vi "control function to channels.vi"(11 "control module configuration":T1 {"output range"."output low" format="%.2f"; "output range"."output high" format="%.2f"}) -> (3 "channels":refnum<class "TBM channel.lvclass">[](array[class]))   [LabVIEW 2013, in "configuration tests.lvlib" / "TEST CONFIGURATION.lvclass"]
uses:
  TEST CONFIGURATION.lvclass
  <vilib>/NI/Tag Bus Module Framework/channel/TBM channel.lvclass
  control module configuration.ctl
  gains.ctl
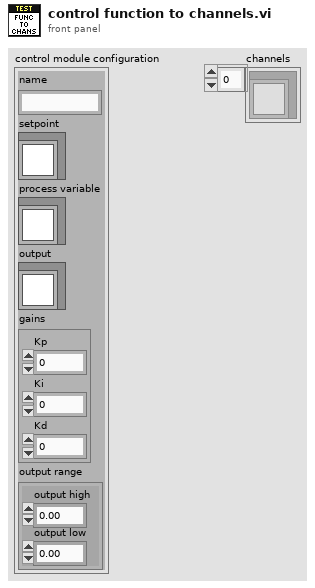
[diagram p1: front panel]
types:
  T1 = typedef "configuration tests.lvlib/TEST CONFIGURATION.lvclass/control module configuration.ctl" = cluster{"name":string, "setpoint":refnum<class "TBM channel.lvclass">, "process variable":refnum<class "TBM channel.lvclass">, "output":refnum<class "TBM channel.lvclass">, "gains":T2, "output range":cluster{"output high":dbl, "output low":dbl}}
  T2 = typedef "configuration tests.lvlib/TEST CONFIGURATION.lvclass/gains.ctl" = cluster{"Kp":dbl, "Ki":dbl, "Kd":dbl}
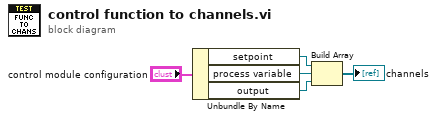
[diagram p0: block diagram]
diagram:
  n1 = Unbundle By Name("control module configuration") -> ("setpoint"=w2:refnum<class "TBM channel.lvclass">, "process variable"=w5:refnum<class "TBM channel.lvclass">, "output"=w4:refnum<class "TBM channel.lvclass">)
  n2 = Build Array(w2, w5, w4) -> (→"channels":refnum<class "TBM channel.lvclass">[])
